vi "ACW Test for MANU.vi"(8 "error in":errorcluster, 11 "VISA resource name":refnum<visa-resource-name>) -> (0 "error out":errorcluster, 3 "VISA resource name out":refnum<visa-resource-name>)   [LabVIEW 2011, in "GPT-9000.lvlib"]
uses:
  <instrlib>/GPT-9000/GPT-9000.lvlib
panel:
  in  "Ground mode Setting":u8(ring) items=["OFF", "ON"]
  in  "ARC mode":u8(ring) items=["OFF", "ON_CONT", "ON_STOP"]
  out "ARC":bool
  out "Ready to Start":bool
  out "Error LED":bool
  out "Time":string
  out "Current":string
  out "Voltage":string
  out "Error Message":string
  out "LED":bool
  out "TEST":bool
  out "READY":bool
  in  "Clear Error(True)":bool=TRUE
  in  "ID Query (True)":bool=TRUE
  out "FAIL":bool
  out "PASS":bool
  out "ID Return String":string
  in  "Start":bool
  in  "Stop":bool
  in  "ACW ARC current value(mA)":sgl=80.0 min=0 max=80 format="%.1f"
  in  "ACW reference value(mA)":sgl min=0 max=41.9 format="%.1f"
  in  "ACW Test Frequency(Hz)":u8(ring)=1 items=["50", "60"]
  in  "ACW Test Time(S)":sgl=1.0 min=0.5 max=999.9 format="%.1f"
  in  "ACW LO SET current value(mA)":sgl min=0 max=41.9 format="%.3f"
  in  "ACW HI SET current value(mA)":sgl=42.0 min=0.001 max=42 format="%.3f"
  in  "ACW voltage(kV)":sgl=1.0 min=0.1 max=5 format="%.3f"
  in  "Ramp Time":sgl=1.0 min=0.1 max=999.9 format="%.1f"
  in  "Test name":string="TEST_NAME"
  in  "Test number":u8 max=100
  in  "Configure RS232 Baud Rate":u32(ring)=115200 items=["9600"=9600, "19200"=19200, "38400"=38400, "57600"=57600, "115200"=115200]
  # "ACW Test for MENU Mode"
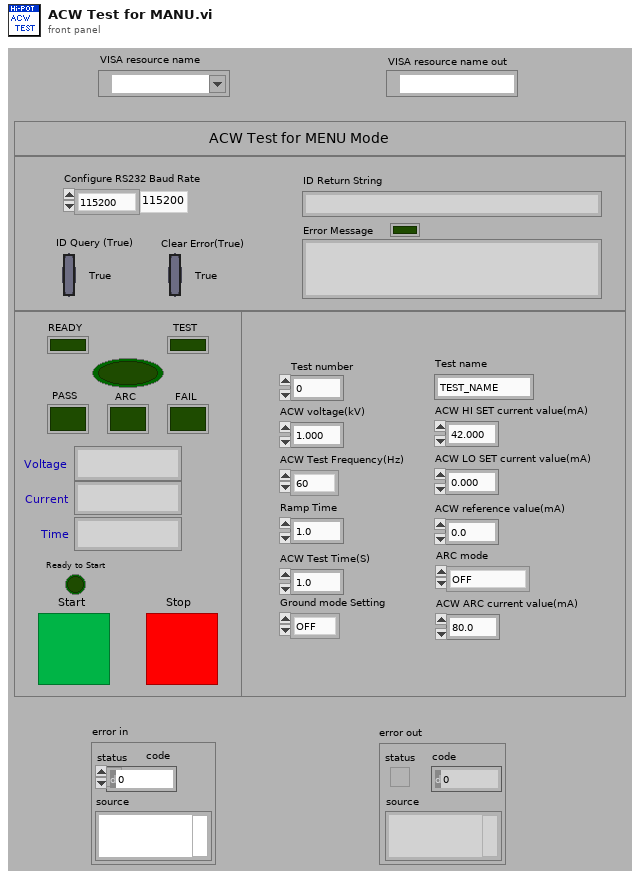
[diagram p1: front panel]
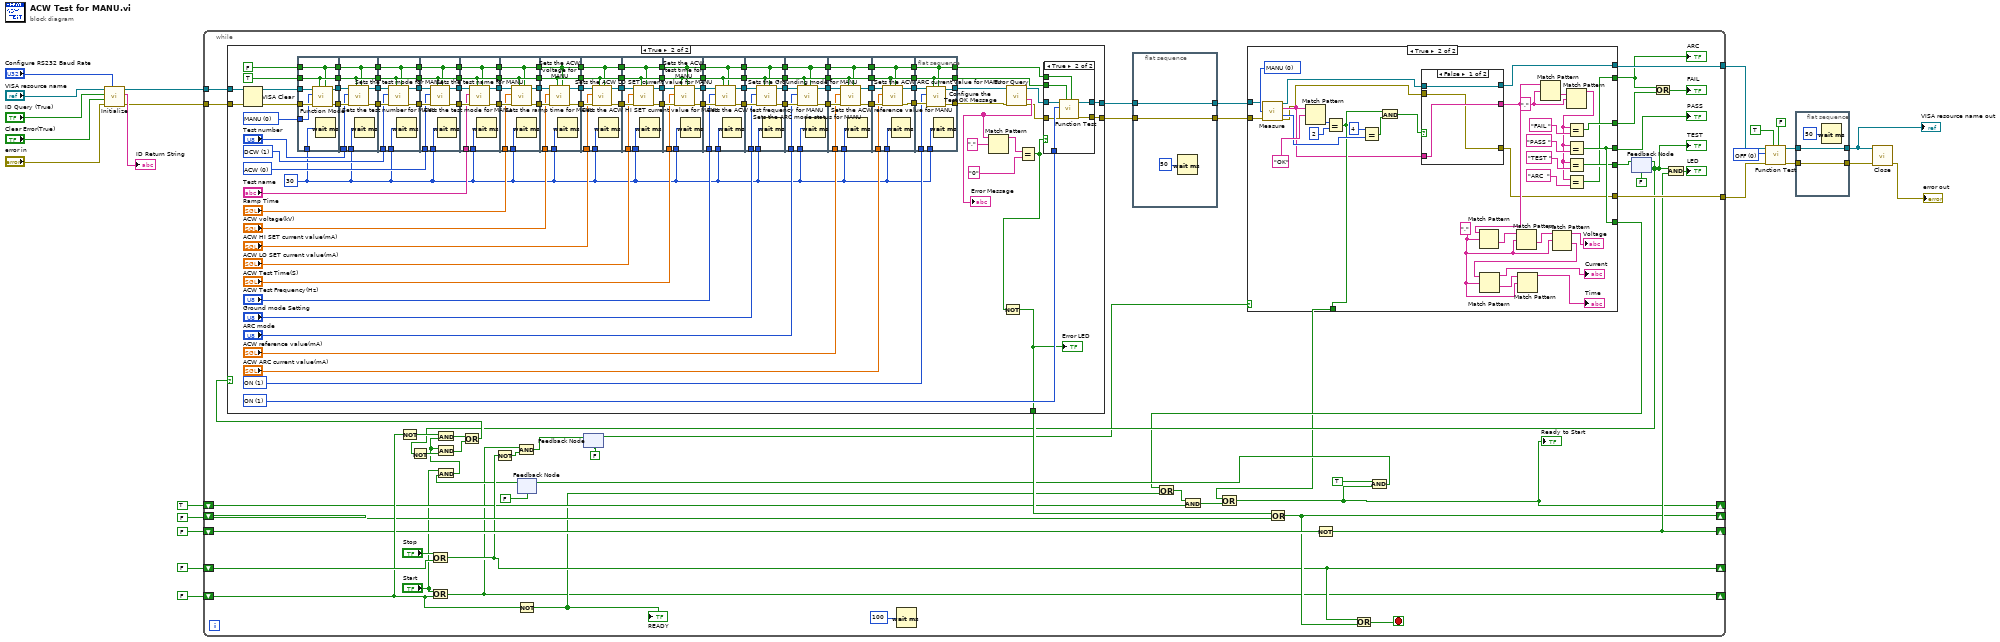
[diagram p0: block diagram]
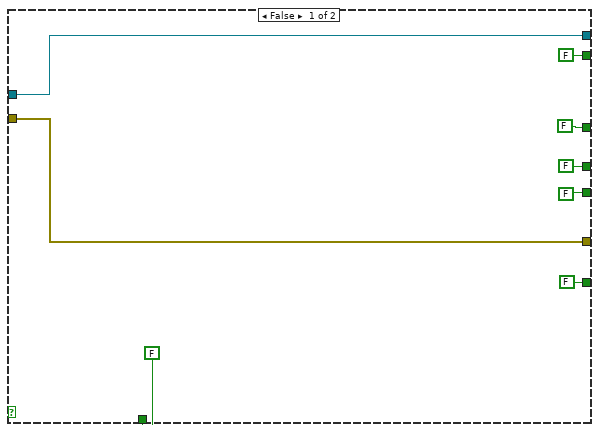
[diagram p2: hidden frame]
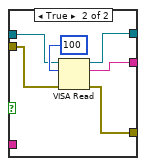
[diagram p3: hidden frame]
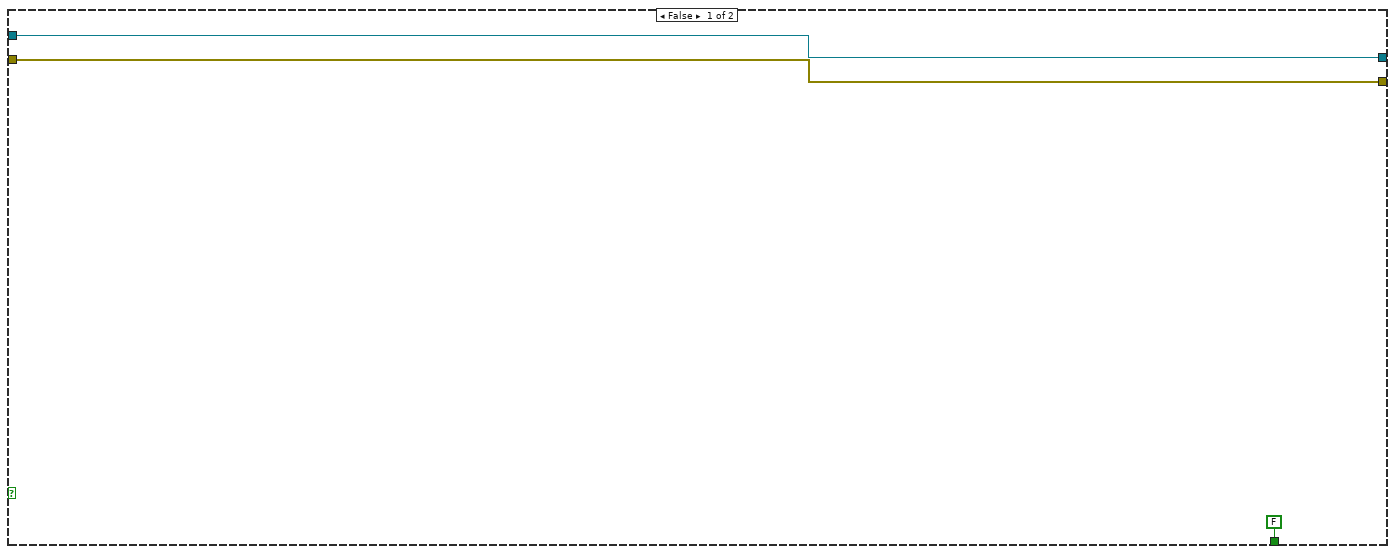
[diagram p4: hidden frame]
diagram:
  w21 = u8 0 items=["OFF", "ON"] ("Function Test")
  n1 = call <instrlib>:"Initialize.vi"("Configure RS232 Baud Rate"="Configure RS232 Baud Rate", "error in (no error)"="error in", "Clear Error(True)"="Clear Error(True)", "ID Query (True)"="ID Query (True)", "VISA resource name"="VISA resource name") -> ("error out"=w10:errorcluster, "ID Return String"=→"ID Return String":string, "VISA resource name out"=w11:refnum<visa-resource-name>)  [unwired: 3 in, 1 out]
  n2 = while {
    shift-right: [w29] -> _
    shift-left: FALSE -> [w66]
    shift-right: [w51] -> _
    shift-left: FALSE -> [w72]
    tunnel: [w71] -> w23
    tunnel: [w70] -> w22
    shift-right: [w65] -> _
    shift-left: FALSE -> [w64]
    tunnel: w11 -> [w58]
    tunnel: w10 -> [w57]
    shift-right: [w54] -> _
    shift-left: FALSE -> [w55]
    shift-right: [w40] -> _
    shift-left: TRUE -> [w45]
    stop <- w56 stop-if-true
    n3 = Not(x=w66) -> (.not. x?=w69:bool)
    n4 = Or(x="Stop", y=w72) -> (x .or. y?=w51:bool)
    n5 = Or(x="Start", y=w66) -> (x .or. y?=w29:bool)
    n6 = Not(x=w51) -> (.not. x?=w68:bool)
    n7 = And(x=w29, y=w68) -> (x .and. y?=w67:bool)
    n8 = feedback #1(FALSE) -> (w38:bool)
    n9 = And(x="Start", y=w38) -> (x .and. y?=w42:bool)
    n10 = And(x=w69, y=w42) -> (x .and. y?=w61:bool)
    n11 = Not(x=w66) -> (.not. x?=w43:bool)
    "READY" <- w43
    n12 = feedback-in #2(w67) -> ()
    n13 = feedback #2(FALSE) -> (w35:bool)
    n14 = Wait (ms)(milliseconds to wait=u32 100) -> ()  [unwired: 1 out]
    n15 = flat-sequence {
      tunnel: [w76] -> w26
      tunnel: w27 -> [w76]
      tunnel: w25 -> [w75]
      tunnel: [w75] -> w24
      frame #0 {
        n16 = Wait (ms)(milliseconds to wait=u32 50) -> ()  [unwired: 1 out]
      }
    }
    n17 = case shown="True" w35 {
      tunnel: [w79 w94] -> w71
      tunnel: [w78 w93] -> w70
      tunnel: [FALSE w105] -> w34
      tunnel: [FALSE w115] -> w31
      tunnel: [FALSE w105] -> w47
      tunnel: [FALSE w104] -> w50
      tunnel: [FALSE w102] -> w30
      tunnel: w26 -> [w79 w100]
      tunnel: w24 -> [w78 w99]
      tunnel: [FALSE w89] -> w28
      frame False {
      }
      frame True {
        w106 = u8 0 items=["MANU", "AUTO"] ("Function Mode Numeric")
        w107 = "," ("regular expression")
        w117 = "," ("regular expression")
        n18 = call <instrlib>:"Measure.vi"("VISA resource name"=w100, "Function Mode Numeric"=w106, "error in"=w99) -> ("VISA resource name out"=w86:refnum<visa-resource-name>, "Return  the test status"=w88:string, "Return the String Count"=w91:u16, "error out"=w85:errorcluster)  [unwired: 9 in]
        n19 = Match Pattern(string=w88, regular expression="OK") -> (offset past match=w97:i32)  [unwired: 1 in, 3 out]
        n20 = Equal?(x=w97, y=2) -> (x = y?=w89:bool)
        n21 = Equal?(x=u16 4, y=w91) -> (x = y?=w92:bool)
        n22 = And(x=w89, y=w92) -> (x .and. y?=w87:bool)
        n23 = case shown="False" w87 {
          tunnel: [w123 w128] -> w94
          tunnel: [w121 w127] -> w93
          tunnel: [w122 w126] -> w95
          tunnel: w86 -> [w123 w125]
          tunnel: w88 -> [w122 _]
          tunnel: w85 -> [w121 w124]
          frame False {
          }
          frame True {
            n24 = VISA Read(VISA resource name=w125, byte count=u32 100, error in (no error)=w124) -> (VISA resource name out=w128:refnum<visa-resource-name>, read buffer=w126:string, error out=w127:errorcluster)  [unwired: 1 out]
          }
        }
        n25 = Match Pattern(string=w95, regular expression=w107) -> (after substring=w114:string)  [unwired: 1 in, 3 out]
        n26 = Match Pattern(string=w114, regular expression=w107) -> (after substring=w110:string)  [unwired: 1 in, 3 out]
        n27 = Match Pattern(string=w95, regular expression=w117) -> (after substring=w118:string)  [unwired: 1 in, 3 out]
        n28 = Match Pattern(string=w110, regular expression=w107) -> (before substring=→"Voltage":string, after substring=w108:string)  [unwired: 1 in, 2 out]
        n29 = Match Pattern(string=w108, regular expression=w107) -> (before substring=→"Current":string, after substring=w113:string)  [unwired: 1 in, 2 out]
        n30 = Match Pattern(string=w113, regular expression=w107) -> (before substring=→"Time":string)  [unwired: 1 in, 3 out]
        n31 = Match Pattern(string=w118, regular expression=w117) -> (before substring=w101:string)  [unwired: 1 in, 3 out]
        n32 = Equal?(x=w101, y="FAIL ") -> (x = y?=w115:bool)
        n33 = Equal?(x=w101, y="PASS ") -> (x = y?=w105:bool)
        n34 = Equal?(x=w101, y="TEST ") -> (x = y?=w104:bool)
        n35 = Equal?(x=w101, y="ARC  ") -> (x = y?=w102:bool)
      }
    }
    "PASS" <- w47
    "ARC" <- w30
    n36 = Or(x=w34, y=w43) -> (x .or. y?=w44:bool)
    n37 = And(x=w44, y=w45) -> (x .and. y?=w46:bool)
    n38 = Or(x=w28, y=w46) -> (x .or. y?=w40:bool)
    "Ready to Start" <- w40
    n39 = Not(x=w64) -> (.not. x?=w65:bool)
    n40 = And(x=TRUE, y=w40) -> (x .and. y?=w36:bool)
    n41 = feedback-in #1(w36) -> ()
    n42 = feedback-in #3(w50) -> ()
    n43 = feedback #3(FALSE) -> (w49:bool)
    "TEST" <- w49
    n44 = Not(x=w49) -> (.not. x?=w59:bool)
    n45 = And(x=w42, y=w59) -> (x .and. y?=w60:bool)
    n46 = Or(x=w61, y=w60) -> (x .or. y?=w52:bool)
    n47 = case shown="True" w52 {
      tunnel: w58 -> [w132 w219]
      tunnel: w57 -> [w131 w218]
      tunnel: [w132 w229] -> w27
      tunnel: [w131 w228] -> w25
      tunnel: [FALSE w222] -> w53
      frame False {
      }
      frame True {
        w133 = u32 30 ("milliseconds to wait")
        w157 = u8 1 items=["ACW", "DCW", "IR", "GB"] ("Test Mode")
        w134 = u8 1 items=["OFF", "ON"] ("Send Message when test stop")
        w156 = u8 0 items=["ACW", "DCW", "IR", "GB"] ("Test Mode")
        w159 = u8 0 items=["AUTO"=1, "MANU"=0] ("Function Mode")
        w230 = u8 1 items=["OFF", "ON"] ("Function Test")
        n48 = VISA Clear(VISA resource name=w219, error in (no error)=w218) -> (VISA resource name out=w217:refnum<visa-resource-name>, error out=w216:errorcluster)
        n49 = flat-sequence {
          tunnel: w217 -> [w238]
          tunnel: w216 -> [w237]
          tunnel: [w236] -> w215
          tunnel: [w235] -> w214
          tunnel: TRUE -> [w234]
          tunnel: [w234] -> w176
          tunnel: FALSE -> [w233]
          tunnel: [w233] -> w161
          tunnel: w159 -> [w232]
          tunnel: w133 -> [w231]
          tunnel: w215 -> [w246]
          tunnel: w214 -> [w245]
          tunnel: [w244] -> w213
          tunnel: [w243] -> w212
          tunnel: [w242] -> w177
          tunnel: w176 -> [w242]
          tunnel: [w241] -> w162
          tunnel: w161 -> [w241]
          tunnel: "Test number" -> [w240]
          tunnel: w133 -> [w239]
          tunnel: w213 -> [w254]
          tunnel: w212 -> [w253]
          tunnel: [w252] -> w211
          tunnel: [w251] -> w210
          tunnel: [w250] -> w178
          tunnel: w177 -> [w250]
          tunnel: [w249] -> w163
          tunnel: w162 -> [w249]
          tunnel: w157 -> [w248]
          tunnel: w133 -> [w247]
          tunnel: w211 -> [w262]
          tunnel: w210 -> [w261]
          tunnel: [w260] -> w209
          tunnel: [w259] -> w208
          tunnel: [w258] -> w179
          tunnel: w178 -> [w258]
          tunnel: [w257] -> w164
          tunnel: w163 -> [w257]
          tunnel: w156 -> [w256]
          tunnel: w133 -> [w255]
          tunnel: w209 -> [w270]
          tunnel: w208 -> [w269]
          tunnel: [w268] -> w207
          tunnel: [w267] -> w206
          tunnel: [w266] -> w180
          tunnel: w179 -> [w266]
          tunnel: [w265] -> w165
          tunnel: w164 -> [w265]
          tunnel: "Test name" -> [w264]
          tunnel: w133 -> [w263]
          tunnel: w207 -> [w278]
          tunnel: w206 -> [w277]
          tunnel: [w276] -> w205
          tunnel: [w275] -> w204
          tunnel: [w274] -> w181
          tunnel: w180 -> [w274]
          tunnel: [w273] -> w166
          tunnel: w165 -> [w273]
          tunnel: "Ramp Time" -> [w272]
          tunnel: w133 -> [w271]
          tunnel: w205 -> [w286]
          tunnel: w204 -> [w285]
          tunnel: [w284] -> w203
          tunnel: [w283] -> w202
          tunnel: [w282] -> w182
          tunnel: w181 -> [w282]
          tunnel: [w281] -> w167
          tunnel: w166 -> [w281]
          tunnel: "ACW voltage(kV)" -> [w280]
          tunnel: w133 -> [w279]
          tunnel: w203 -> [w294]
          tunnel: w202 -> [w293]
          tunnel: [w292] -> w201
          tunnel: [w291] -> w200
          tunnel: [w290] -> w183
          tunnel: w182 -> [w290]
          tunnel: [w289] -> w168
          tunnel: w167 -> [w289]
          tunnel: "ACW HI SET current value(mA)" -> [w288]
          tunnel: w133 -> [w287]
          tunnel: w201 -> [w302]
          tunnel: w200 -> [w301]
          tunnel: [w300] -> w199
          tunnel: [w299] -> w198
          tunnel: [w298] -> w184
          tunnel: w183 -> [w298]
          tunnel: [w297] -> w169
          tunnel: w168 -> [w297]
          tunnel: "ACW LO SET current value(mA)" -> [w296]
          tunnel: w133 -> [w295]
          tunnel: w199 -> [w310]
          tunnel: w198 -> [w309]
          tunnel: [w308] -> w197
          tunnel: [w307] -> w196
          tunnel: [w306] -> w185
          tunnel: w184 -> [w306]
          tunnel: [w305] -> w170
          tunnel: w169 -> [w305]
          tunnel: "ACW Test Time(S)" -> [w304]
          tunnel: w133 -> [w303]
          tunnel: w197 -> [w318]
          tunnel: w196 -> [w317]
          tunnel: [w316] -> w195
          tunnel: [w315] -> w194
          tunnel: [w314] -> w186
          tunnel: w185 -> [w314]
          tunnel: [w313] -> w171
          tunnel: w170 -> [w313]
          tunnel: "ACW Test Frequency(Hz)" -> [w312]
          tunnel: w133 -> [w311]
          tunnel: w195 -> [w326]
          tunnel: w194 -> [w325]
          tunnel: [w324] -> w193
          tunnel: [w323] -> w192
          tunnel: [w322] -> w187
          tunnel: w186 -> [w322]
          tunnel: [w321] -> w172
          tunnel: w171 -> [w321]
          tunnel: "Ground mode Setting" -> [w320]
          tunnel: w133 -> [w319]
          tunnel: w193 -> [w334]
          tunnel: w192 -> [w333]
          tunnel: [w332] -> w191
          tunnel: [w331] -> w190
          tunnel: [w330] -> w188
          tunnel: w187 -> [w330]
          tunnel: [w329] -> w173
          tunnel: w172 -> [w329]
          tunnel: "ARC mode" -> [w328]
          tunnel: w133 -> [w327]
          tunnel: w191 -> [w342]
          tunnel: w190 -> [w341]
          tunnel: w188 -> [w338]
          tunnel: w173 -> [w337]
          tunnel: "ACW reference value(mA)" -> [w336]
          tunnel: w133 -> [w335]
          tunnel: [w340] -> w145
          tunnel: [w339] -> w144
          tunnel: [w338] -> w143
          tunnel: [w337] -> w142
          tunnel: w145 -> [w350]
          tunnel: w144 -> [w348]
          tunnel: w143 -> [w344]
          tunnel: w142 -> [w343]
          tunnel: "ACW ARC current value(mA)" -> [w346]
          tunnel: w133 -> [w345]
          tunnel: [w344] -> w140
          tunnel: [w343] -> w139
          tunnel: [w349] -> w138
          tunnel: [w347] -> w137
          tunnel: [w352] -> w160
          tunnel: [w353] -> w175
          tunnel: w140 -> [w353]
          tunnel: w139 -> [w352]
          tunnel: w138 -> [w357]
          tunnel: w137 -> [w356]
          tunnel: [w355] -> w136
          tunnel: [w354] -> w135
          tunnel: w134 -> [w351]
          tunnel: w133 -> [w358]
          frame #0 {
            n50 = call <instrlib>:"Function Mode.vi"("Enable to Query"=w233, "Enable to Setup"=w234, "error in"=w237, "Function Mode"=w232, "VISA resource name"=w238) -> ("error out"=w235:errorcluster, "VISA resource name out"=w236:refnum<visa-resource-name>)  [unwired: 4 in, 1 out]
            n51 = Wait (ms)(milliseconds to wait=w231) -> ()  [unwired: 1 out]
          }
          frame #1 {
            n52 = call <instrlib>:"Sets the test number for MANU.vi"("Enable to Query"=w241, "Enable to Setup"=w242, "error in"=w245, "Test number"=w240, "VISA resource name"=w246) -> ("error out"=w243:errorcluster, "VISA resource name out"=w244:refnum<visa-resource-name>)  [unwired: 4 in, 1 out]
            n53 = Wait (ms)(milliseconds to wait=w239) -> ()  [unwired: 1 out]
          }
          frame #2 {
            n54 = call <instrlib>:"Sets the test mode for MANU.vi"("Enable to Query"=w249, "Enable to Setup"=w250, "error in"=w253, "Test Mode"=w248, "VISA resource name"=w254) -> ("error out"=w251:errorcluster, "VISA resource name out"=w252:refnum<visa-resource-name>)  [unwired: 4 in, 1 out]
            n55 = Wait (ms)(milliseconds to wait=w247) -> ()  [unwired: 1 out]
          }
          frame #3 {
            n56 = call <instrlib>:"Sets the test mode for MANU.vi"("Enable to Query"=w257, "Enable to Setup"=w258, "error in"=w261, "Test Mode"=w256, "VISA resource name"=w262) -> ("error out"=w259:errorcluster, "VISA resource name out"=w260:refnum<visa-resource-name>)  [unwired: 4 in, 1 out]
            n57 = Wait (ms)(milliseconds to wait=w255) -> ()  [unwired: 1 out]
          }
          frame #4 {
            n58 = call <instrlib>:"Sets the test name for MANU.vi"("Enable to Query"=w265, "Enable to Setup"=w266, "error in"=w269, "Test name"=w264, "VISA resource name"=w270) -> ("error out"=w267:errorcluster, "VISA resource name out"=w268:refnum<visa-resource-name>)  [unwired: 4 in, 1 out]
            n59 = Wait (ms)(milliseconds to wait=w263) -> ()  [unwired: 1 out]
          }
          frame #5 {
            n60 = call <instrlib>:"Sets the ramp time for MANU.vi"("Enable to Query"=w273, "Enable to Setup"=w274, "error in"=w277, "Ramp Time"=w272, "VISA resource name"=w278) -> ("error out"=w275:errorcluster, "VISA resource name out"=w276:refnum<visa-resource-name>)  [unwired: 4 in, 1 out]
            n61 = Wait (ms)(milliseconds to wait=w271) -> ()  [unwired: 1 out]
          }
          frame #6 {
            n62 = call <instrlib>:"Sets the ACW voltage for MANU.vi"("Enable to Query"=w281, "Enable to Setup"=w282, "error in"=w285, "ACW voltage(kV)"=w280, "VISA resource name"=w286) -> ("error out"=w283:errorcluster, "VISA resource name out"=w284:refnum<visa-resource-name>)  [unwired: 4 in, 1 out]
            n63 = Wait (ms)(milliseconds to wait=w279) -> ()  [unwired: 1 out]
          }
          frame #7 {
            n64 = call <instrlib>:"Sets the ACW HI SET current value for MANU.vi"("Enable to Query"=w289, "Enable to Setup"=w290, "error in"=w293, "ACW HI SET current value(mA)"=w288, "VISA resource name"=w294) -> ("error out"=w291:errorcluster, "VISA resource name out"=w292:refnum<visa-resource-name>)  [unwired: 4 in, 1 out]
            n65 = Wait (ms)(milliseconds to wait=w287) -> ()  [unwired: 1 out]
          }
          frame #8 {
            n66 = call <instrlib>:"Sets the ACW LO SET current value for MANU.vi"("Enable to Query"=w297, "Enable to Setup"=w298, "error in"=w301, "ACW LO SET current value(mA)"=w296, "VISA resource name"=w302) -> ("error out"=w299:errorcluster, "VISA resource name out"=w300:refnum<visa-resource-name>)  [unwired: 4 in, 1 out]
            n67 = Wait (ms)(milliseconds to wait=w295) -> ()  [unwired: 1 out]
          }
          frame #9 {
            n68 = call <instrlib>:"Sets the ACW test time for MANU.vi"("Enable to Query"=w305, "Enable to Setup"=w306, "error in"=w309, "ACW Test Time(S)"=w304, "VISA resource name"=w310) -> ("error out"=w307:errorcluster, "VISA resource name out"=w308:refnum<visa-resource-name>)  [unwired: 4 in, 1 out]
            n69 = Wait (ms)(milliseconds to wait=w303) -> ()  [unwired: 1 out]
          }
          frame #10 {
            n70 = call <instrlib>:"Sets the ACW test frequency for MANU.vi"("Enable to Query"=w313, "Enable to Setup"=w314, "error in"=w317, "ACW Test Frequency(Hz)"=w312, "VISA resource name"=w318) -> ("error out"=w315:errorcluster, "VISA resource name out"=w316:refnum<visa-resource-name>)  [unwired: 4 in, 1 out]
            n71 = Wait (ms)(milliseconds to wait=w311) -> ()  [unwired: 1 out]
          }
          frame #11 {
            n72 = call <instrlib>:"Sets the Grounding mode for MANU.vi"("Enable to Query the Ground mode"=w321, "Enable to Setup the Ground mode"=w322, "error in"=w325, "Ground mode Setting"=w320, "VISA resource name"=w326) -> ("error out"=w323:errorcluster, "VISA resource name out"=w324:refnum<visa-resource-name>)  [unwired: 4 in, 1 out]
            n73 = Wait (ms)(milliseconds to wait=w319) -> ()  [unwired: 1 out]
          }
          frame #12 {
            n74 = call <instrlib>:"Sets the ARC mode status for MANU.vi"("Enable to Query the ARC mode"=w329, "Enable to Setup the ARC mode"=w330, "error in"=w333, "ARC mode"=w328, "VISA resource name"=w334) -> ("error out"=w331:errorcluster, "VISA resource name out"=w332:refnum<visa-resource-name>)  [unwired: 4 in, 1 out]
            n75 = Wait (ms)(milliseconds to wait=w327) -> ()  [unwired: 1 out]
          }
          frame #13 {
            n76 = call <instrlib>:"Sets the ACW reference value for MANU.vi"("Enable to Query"=w337, "Enable to Setup"=w338, "error in"=w341, "ACW reference value(mA)"=w336, "VISA resource name"=w342) -> ("error out"=w339:errorcluster, "VISA resource name out"=w340:refnum<visa-resource-name>)  [unwired: 4 in, 1 out]
            n77 = Wait (ms)(milliseconds to wait=w335) -> ()  [unwired: 1 out]
          }
          frame #14 {
            n78 = call <instrlib>:"Sets the ACW ARC current value for MANU.vi"("Enable to Query"=w343, "Enable to Setup"=w344, "error in"=w348, "ACW ARC current value(mA)"=w346, "VISA resource name"=w350) -> ("error out"=w347:errorcluster, "VISA resource name out"=w349:refnum<visa-resource-name>)  [unwired: 4 in, 1 out]
            n79 = Wait (ms)(milliseconds to wait=w345) -> ()  [unwired: 1 out]
          }
          frame #15 {
            n80 = call <instrlib>:"Configure the Test OK Message.vi"("Query the Message"=w352, "Setup the Message"=w353, "error in"=w356, "Send Message when test stop"=w351, "VISA resource name"=w357) -> ("error out"=w354:errorcluster, "VISA resource name out"=w355:refnum<visa-resource-name>)  [unwired: 4 in, 1 out]
            n81 = Wait (ms)(milliseconds to wait=w358) -> ()  [unwired: 1 out]
          }
        }
        n82 = call <instrlib>:"Error Query.vi"("error in (no error)"=w135, "VISA resource name"=w136) -> ("error out"=w221:errorcluster, "Error Message"=w224:string, "VISA resource name out"=w220:refnum<visa-resource-name>)  [unwired: 6 in, 1 out]
        "Error Message" <- w224
        n83 = Match Pattern(string=w224, regular expression=",") -> (before substring=w226:string)  [unwired: 1 in, 3 out]
        n84 = Equal?(x=w226, y="0") -> (x = y?=w223:bool)
        n85 = Not(x=w223) -> (.not. x?=w222:bool)
        "Error LED" <- w222
        n86 = case shown="True" w223 {
          tunnel: w230 -> [_ w367]
          tunnel: w220 -> [w360 w366]
          tunnel: w221 -> [w359 w365]
          tunnel: [w360 w364] -> w229
          tunnel: [w359 w363] -> w228
          tunnel: w175 -> [_ w362]
          tunnel: w160 -> [_ w361]
          frame False {
          }
          frame True {
            n87 = call <instrlib>:"Function Test.vi"("VISA resource name"=w366, "Function Test"=w367, "error in"=w365, "Enable to Setup"=w362, "Enable to Query"=w361) -> ("VISA resource name out"=w364:refnum<visa-resource-name>, "error out"=w363:errorcluster)  [unwired: 3 in, 1 out]
          }
        }
      }
    }
    n88 = Or(x=w53, y=w55) -> (x .or. y?=w54:bool)
    n89 = Or(x=w51, y=w54) -> (x .or. y?=w56:bool)
    n90 = Or(x=w30, y=w31) -> (x .or. y?=→"FAIL":bool)
    n91 = And(x=w49, y=w65) -> (x .and. y?=→"LED":bool)
  }
  n92 = call <instrlib>:"Function Test.vi"("VISA resource name"=w23, "Function Test"=w21, "error in"=w22, "Enable to Setup"=TRUE, "Enable to Query"=FALSE) -> ("VISA resource name out"=w5:refnum<visa-resource-name>, "error out"=w3:errorcluster)  [unwired: 3 in, 1 out]
  n93 = flat-sequence {
    tunnel: w5 -> [w370]
    tunnel: [w370] -> w4
    tunnel: w3 -> [w369]
    tunnel: [w369] -> w2
    frame #0 {
      n94 = Wait (ms)(milliseconds to wait=u32 50) -> ()  [unwired: 1 out]
    }
  }
  n95 = call <instrlib>:"Close.vi"("error in (no error)"=w2, "VISA resource name"=w4) -> ("error out"=→"error out":errorcluster)  [unwired: 9 in]
  "VISA resource name out" <- w4
